vi "Feenstra type spectroscopy.vi"() -> ()   [LabVIEW 2017]
doc: "<B>Feenstra type spectroscopy</B>\nThis VI performs a Feenstra type spectroscopy measurement. See front panel for more details.\n\n- Nanonis Programming Interface -"
uses:
  Nanonis Prog Interface.lvlib
panel:
  out "error out":errorcluster
  out "z0 (m)":dbl format="%#_5p"
  in  "a+ (m/V)":dbl=1e-10 format="%#_3p"
  out "dV (V)":dbl format="%#_5p"
  out "Z vs Bias":cluster{dbl[], dbl[]}(graph)
  out "Current vs Bias":cluster{dbl[], sgl[]}(graph)
  out "V1 (V)":sgl format="%_3p"
  out "z1 (m)":sgl format="%#_5p"
  in  "no of points for the sweep":i32=51 format="%#.3p"
  in  "Vmax (V)":dbl=2.0 format="%#_3p"
  in  "Vmin (V)":dbl=-2.0 format="%#_3p"
  in  "a- (m/V)":dbl=1e-10 format="%#_6p"
  # "Example VI: Feenstra type spectroscopy\nThis VI performs a Feenstra type spectroscopy measurement (according to \"Tunneling Spectroscopy of the (110) surface of direct-gap III-V semiconductors\", R.M. Feenstra, Physical Review B, Vol 50, Number 7, 15 August 1994-I).\nThe a parameters define the z vs V curve according to z(V) = z0 + a |V| with z0 = z(0). a can be different for positive (a+) and negative (a-) Bias.\nFrom the starting point (V1, z1) we calculate z0 based on the above formula.\nThen a sweep is performed from Vmin to Vmax, adjusting z according to the above formula."
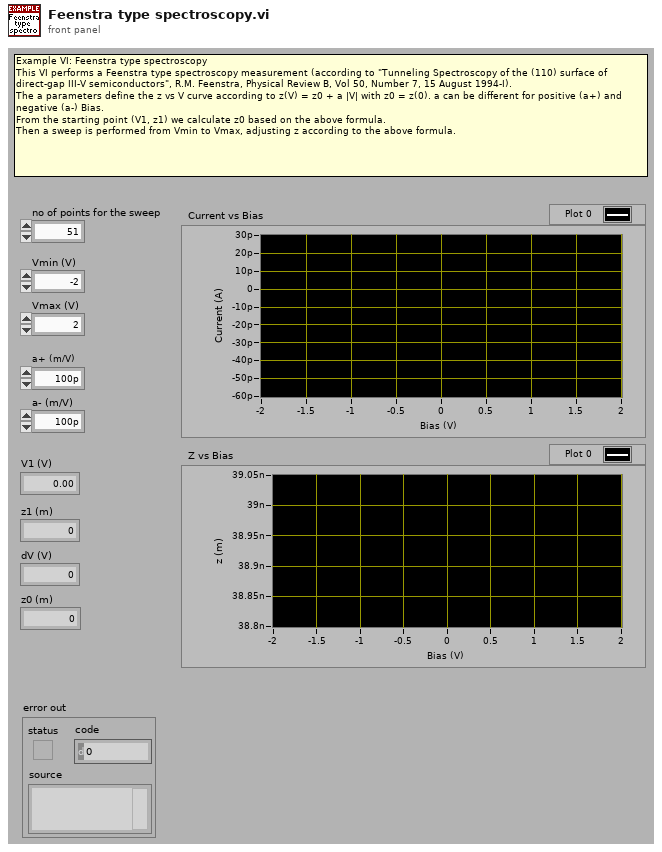
[diagram p1: front panel]
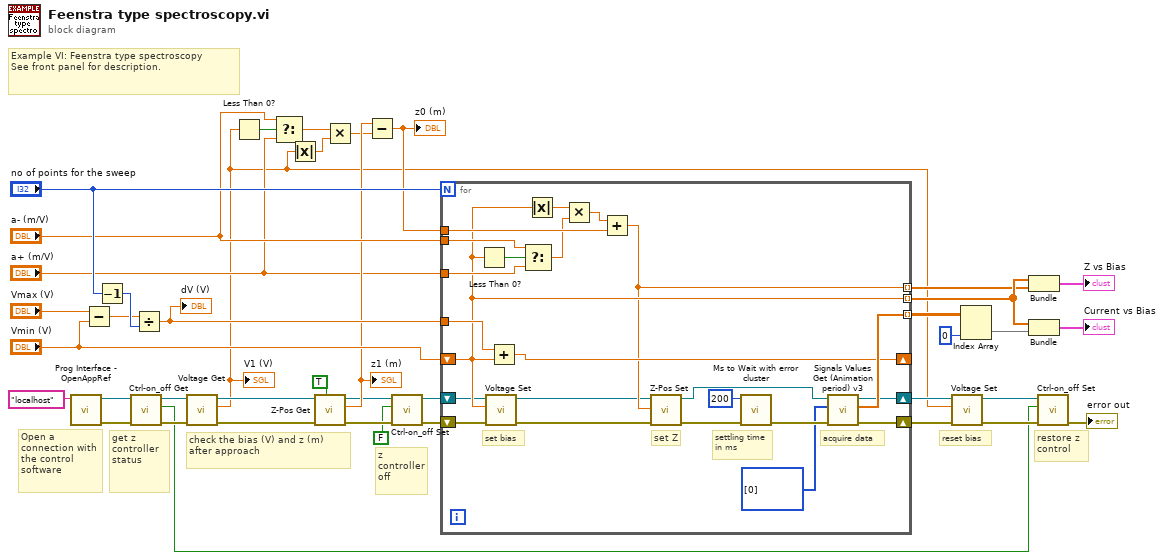
[diagram p0: block diagram]
diagram:
  # "Example VI: Feenstra type spectroscopy\nSee front panel for description."
  # "restore z control"
  # "reset bias"
  # "z controller off"
  # "check the bias (V) and z (m)  after approach"
  # "get z controller status"
  # "Open a connection with the control\nsoftware"
  n1 = call <userlib>:"Prog Interface - OpenAppRef.vi"("Machine name (local machine IP)"="localhost" ("Machine name (localhost)")) -> ("Error out"=w38:errorcluster, "Application reference"=w10:refnum<vi>)  [unwired: 5 in]
  n2 = Subtract(x="Vmax (V)", y="Vmin (V)") -> (x-y=w27:dbl)
  n3 = Decrement(x="no of points for the sweep") -> (x-1=w28:i32)
  n4 = call <userlib>:"Ctrl-on_off Get.vi"("error in (no error)"=w38, "Application ref in"=w10) -> ("error out"=w40:errorcluster, "Z-Controller on/off status"=w11:bool, "Application ref out"=w9:refnum<vi>)  [unwired: 7 in]
  n5 = Divide(x=w27, y=w28) -> (x/y=w23:dbl)
  "dV (V)" <- w23
  n6 = call <userlib>:"Voltage Get.vi"("error in (no error)"=w40, "Application ref in"=w9) -> ("error out"=w39:errorcluster, "Bias (V)"=w3:sgl, "Application ref out"=w8:refnum<vi>)  [unwired: 7 in]
  "V1 (V)" <- w3
  n7 = Less Than 0?(x=w3) -> (x < 0?=w19:bool)
  n8 = Select(t="a- (m/V)", s=w19, f="a+ (m/V)") -> (s? t:f=w17:dbl)
  n9 = Absolute Value(x=w3) -> (abs(x)=w16:sgl)
  n10 = call <userlib>:"Z-Pos Get.vi"("Wait for newest data (F=False)"=TRUE, "error in (no error)"=w39, "Application ref in"=w8) -> ("error out"=w37:errorcluster, "Z position (m)"=w15:sgl, "Application ref out"=w7:refnum<vi>)  [unwired: 6 in]
  "z1 (m)" <- w15
  n11 = Multiply(x=w17, y=w16) -> (x*y=w14:dbl)
  n12 = Subtract(x=w15, y=w14) -> (x-y=w13:dbl)
  "z0 (m)" <- w13
  n13 = call <userlib>:"Ctrl-on_off Set.vi"("error in (no error)"=w37, "Z Controller ON/OFF"=FALSE, "Application ref in"=w7) -> ("error out"=w36:errorcluster, "Application ref out"=w6:refnum<vi>)  [unwired: 7 in]
  n14 = for {
    N: "no of points for the sweep" -> [_]
    tunnel: "a- (m/V)" -> [w51]
    tunnel: w13 -> [w62]
    shift-right: [w57] -> w30
    shift-left: w36 -> [w64]
    tunnel: [w56] -> w20 mode=indexing
    shift-right: [w54] -> _
    shift-left: "Vmin (V)" -> [w49]
    tunnel: [w49] -> w32 mode=indexing
    tunnel: [w47] -> w31 mode=indexing
    tunnel: w23 -> [w55]
    tunnel: "a+ (m/V)" -> [w50]
    shift-right: [w42] -> w5
    shift-left: w6 -> [w45]
    # "acquire data"
    # "settling time\nin ms"
    # "set Z"
    # "set bias"
    n15 = Less Than 0?(x=w49) -> (x < 0?=w52:bool)
    n16 = call <userlib>:"Voltage Set.vi"("Error in (no error)"=w64, "Bias (V)"=w49, "Application ref in"=w45) -> ("Error out"=w46:errorcluster, "Application ref out"=w44:refnum<vi>)  [unwired: 7 in]
    n17 = Add(x=w55, y=w49) -> (x+y=w54:dbl)
    n18 = Select(t=w51, s=w52, f=w50) -> (s? t:f=w48:dbl)
    n19 = Absolute Value(x=w49) -> (abs(x)=w63:dbl)
    n20 = Multiply(x=w63, y=w48) -> (x*y=w61:dbl)
    n21 = Add(x=w61, y=w62) -> (x+y=w47:dbl)
    n22 = call <userlib>:"Z-Pos Set.vi"("error in (no error)"=w46, "Z position (m)"=w47, "Application ref in"=w44) -> ("error out"=w59:errorcluster, "Application ref out"=w43:refnum<vi>)  [unwired: 7 in]
    n23 = call "Ms to Wait with error cluster.vi"("error in (no error)"=w59, "milliseconds to wait"=u32 200) -> ("error out"=w58:errorcluster)  [unwired: 4 in, 1 out]
    n24 = call <userlib>:"Signals Values Get (Animation period) v3.vi"("error in (no error)"=w58, "Signals indexes (0-127)"=i8[] [0] ("Signals indexes (0-23)"), "Application ref in"=w43) -> ("error out"=w57:errorcluster, "Signals Values"=w56:sgl[], "Application ref out"=w42:refnum<vi>)  [unwired: 5 in]
  }
  n25 = call <userlib>:"Voltage Set.vi"("Error in (no error)"=w30, "Bias (V)"=w3, "Application ref in"=w5) -> ("Error out"=w29:errorcluster, "Application ref out"=w4:refnum<vi>)  [unwired: 7 in]
  n26 = Index Array(array=w20, index (col)=0 ("disabled index (col)")) -> (element=w21:sgl[])  [unwired: 1 in]
  n27 = Bundle(w32, w31) -> (→"Z vs Bias":cluster{dbl[], dbl[]})  [unwired: 1 in]
  n28 = Bundle(w32, "Signals Values"=w21) -> (→"Current vs Bias":cluster{dbl[], "Signals Values":sgl[]})  [unwired: 1 in]
  n29 = call <userlib>:"Ctrl-on_off Set.vi"("error in (no error)"=w29, "Z Controller ON/OFF"=w11, "Application ref in"=w4) -> ("error out"=→"error out":errorcluster)  [unwired: 7 in, 1 out]
